vi "16_SynchronizedMeasurements.vi"() -> ()   [LabVIEW 2014]
uses:
  SwabianInstruments.TimeTagger
panel:
  out "FileWriter files":string[](array[string])
  out "First timestamp\ndifference":dbl[unit] format="%#.2g"
  out "Time-tag display":T1(graph)
  out "all time-tags\nidentical?":bool
  in  "Start synchronously if available":bool=TRUE
  in  "Use SynchronizedMeasurements":bool=TRUE
  # "This example demonstrates the SynchronizedMeasurements class. The time-tag stream is investigated by a TimeTagStream measurement and simultaneously dumped by a FileWriter measurement. Afterward, the resulting time-tag streams are compared.\n\nSynchronizedMeasurements ensures that both sub-measurements, TimeTagStream and FileWriter, process the very same set of time-tags. It can be activated/deactivated by the \"Use SynchronizedMeasurements\" control. Even with SynchronizedMeasurements, the sub-measurements can be controlled individually (use \"start synchronously if available\" to toggle behavior.\n\nSynchronizedMeasurements has an important impact on the FileWriter: It deactivates the autostart behavior. Without SynchronizedMeasurements, autostart + startFor results in two FileWriter data files, dump.1.ttbin and dump.2.ttbin."
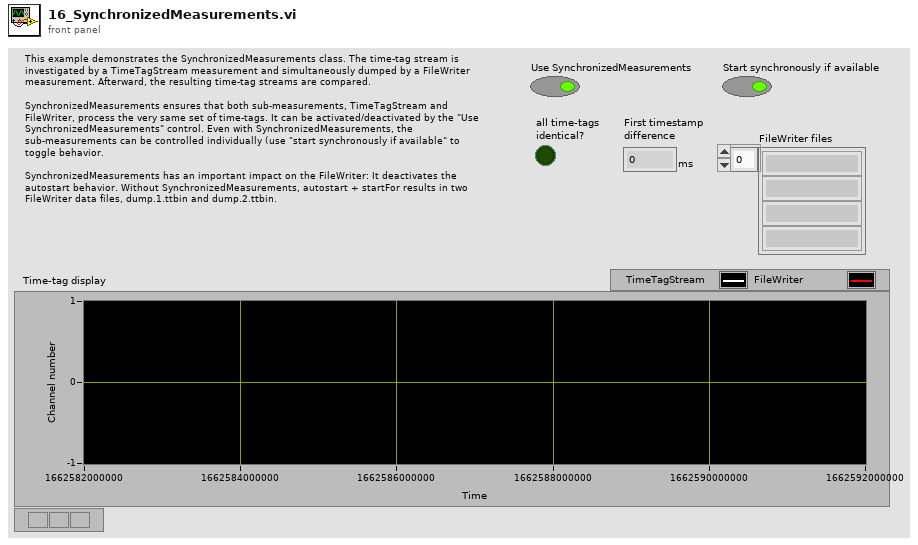
[diagram p1: front panel]
types:
  T1 = cluster{"getTimestamps":i64[], "getChannels":i32[]}[]
  T2 = cluster{"getTimestamps":i64[], "getChannels":i32[]}
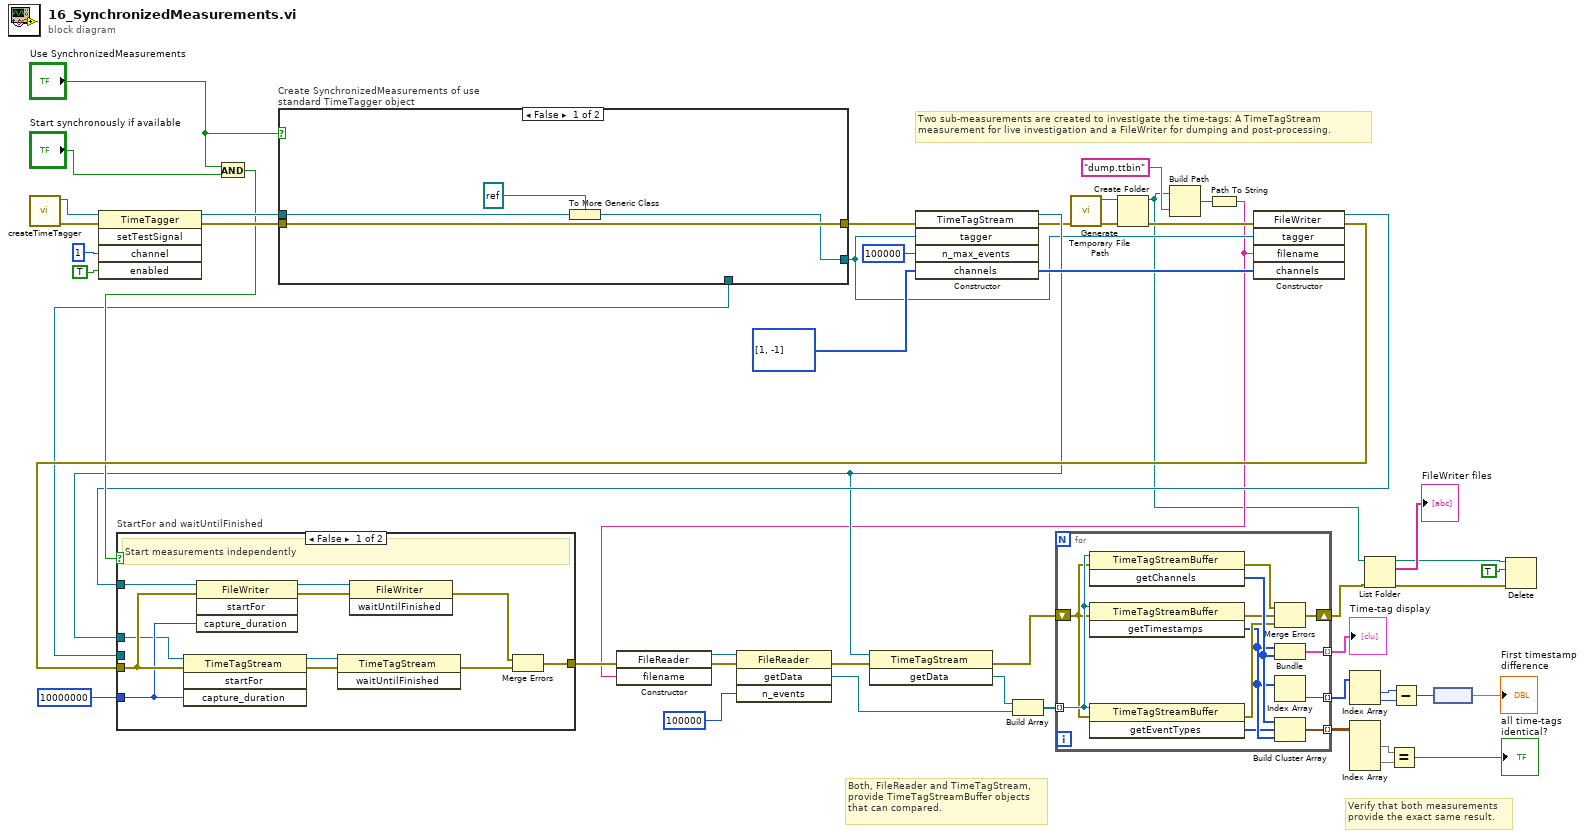
[diagram p0: block diagram]
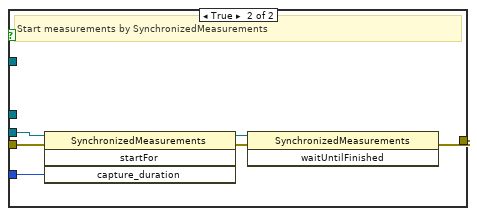
[diagram p2: hidden frame]
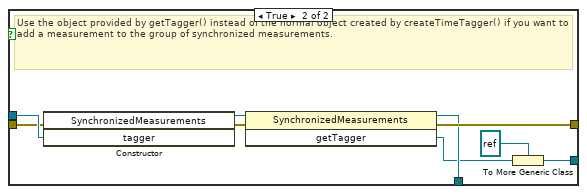
[diagram p3: hidden frame]
diagram:
  # "Both, FileReader and TimeTagStream,\nprovide TimeTagStreamBuffer objects\nthat can compared."
  # "Verify that both measurements\nprovide the exact same result."
  # "Two sub-measurements are created to investigate the time-tags: A TimeTagStream\nmeasurement for live investigation and a FileWriter for dumping and post-processing."
  n1 = call "createTimeTagger.vi"() -> ("error out"=w45:errorcluster, "TimeTagger ref out"=w46:refnum<k24>)  [unwired: 10 in]
  n2 = invoke class="TimeTagger" method="setTestSignal"(reference=w46, error in=w45, "channel"=1, "enabled"=TRUE) -> (reference out=w49:refnum<k24>, error out=w48:errorcluster)  [unwired: 1 in, 3 out]
  n3 = And(x="Use SynchronizedMeasurements", y="Start synchronously if available") -> (x .and. y?=w43:bool)
  n4 = case "Create SynchronizedMeasurements of use standard TimeTagger object" shown="False" "Use SynchronizedMeasurements" {
    tunnel: [w52 w56] -> w14
    tunnel: [w55 w62] -> w50
    tunnel: w49 -> [w53 w61]
    tunnel: w48 -> [w55 w60]
    tunnel: [_ w59] -> w22
    frame False {
      n5 = To More Generic Class(target class=refnum<k24> refnum, reference=w53) -> (generic class reference=w52:refnum<k24>)
    }
    frame True {
      # "Use the object provided by getTagger() instead of the normal object created by createTimeTagger() if you want to add a measurement to the group of synchronized measurements."
      n6 = constructor class="SynchronizedMeasurements"(error in=w60, "tagger"=w61) -> (reference out=w64:refnum<k24>, error out=w63:errorcluster)  [unwired: 2 in, 2 out]
      n7 = invoke class="SynchronizedMeasurements" method="getTagger"(reference=w64, error in=w63) -> (reference out=w59:refnum<k24>, error out=w62:errorcluster, "getTagger"=w58:refnum<k24>)  [unwired: 1 in]
      n8 = To More Generic Class(target class=refnum<k24> refnum, reference=w58) -> (generic class reference=w56:refnum<k24>)
    }
  }
  n9 = constructor class="TimeTagStream"(error in=w50, "tagger"=w14, "n_max_events"=u64 100000, "channels"=i32[] [1, -1]) -> (reference out=w20:refnum<k24>, error out=w5:errorcluster, "channels"=w23:i32[])  [unwired: 2 in, 3 out]
  n10 = call <vilib>:"Generate Temporary File Path.vi"("error in (no error)"=w5) -> ("error out"=w7:errorcluster, "Unique Temporary File Path"=w6:path)  [unwired: 9 in]
  n11 = Create Folder(path (use dialog)=w6, error in=w7) -> (created path=w1:path, error out=w4:errorcluster)  [unwired: 1 in, 1 out]
  n12 = Build Path(base path=w1, name or relative path="dump.ttbin") -> (appended path=w3:path)
  n13 = Path To String(path=w3) -> (string=w2:string)
  n14 = constructor class="FileWriter"(error in=w4, "tagger"=w14, "filename"=w2, "channels"=w23) -> (reference out=w41:refnum<k24>, error out=w47:errorcluster)  [unwired: 2 in, 4 out]
  n15 = case "StartFor and waitUntilFinished" shown="False" w43 {
    tunnel: w47 -> [w71 w81]
    tunnel: w22 -> [_ w80]
    tunnel: [w67 w77] -> w18
    tunnel: i64 10000000 ("capture_duration") -> [w70 w76]
    tunnel: w20 -> [w65 _]
    tunnel: w41 -> [w66 _]
    frame False {
      # "Start measurements independently"
      n16 = invoke class="TimeTagStream" method="startFor"(reference=w65, error in=w71, "capture_duration"=w70) -> (reference out=w73:refnum<k24>, error out=w72:errorcluster)  [unwired: 1 in, 2 out]
      n17 = invoke class="FileWriter" method="startFor"(reference=w66, error in=w71, "capture_duration"=w70) -> (reference out=w75:refnum<k24>, error out=w74:errorcluster)  [unwired: 1 in, 2 out]
      n18 = invoke class="TimeTagStream" method="waitUntilFinished"(reference=w73, error in=w72) -> (error out=w68:errorcluster)  [unwired: 1 in, 2 out]
      n19 = invoke class="FileWriter" method="waitUntilFinished"(reference=w75, error in=w74) -> (error out=w69:errorcluster)  [unwired: 1 in, 2 out]
      n20 = Merge Errors(w69, w68) -> (w67:errorcluster)
    }
    frame True {
      # "Start measurements by SynchronizedMeasurements"
      n21 = invoke class="SynchronizedMeasurements" method="startFor"(reference=w80, error in=w81, "capture_duration"=w76) -> (reference out=w79:refnum<k24>, error out=w78:errorcluster)  [unwired: 1 in, 2 out]
      n22 = invoke class="SynchronizedMeasurements" method="waitUntilFinished"(reference=w79, error in=w78) -> (error out=w77:errorcluster)  [unwired: 1 in, 2 out]
    }
  }
  n23 = constructor class="FileReader"(error in=w18, "filename"=w2) -> (reference out=w40:refnum<k24>, error out=w39:errorcluster)  [unwired: 2 in, 2 out]
  n24 = invoke class="FileReader" method="getData"(reference=w40, error in=w39, "n_events"=u64 100000) -> (error out=w16:errorcluster, "getData"=w31:refnum<k24>)  [unwired: 1 in, 2 out]
  n25 = invoke class="TimeTagStream" method="getData"(reference=w20, error in=w16) -> (error out=w15:errorcluster, "getData"=w38:refnum<k24>)  [unwired: 1 in, 1 out]
  n26 = Build Array(w38, w31) -> (w37:refnum<k24>[])
  n27 = for {
    tunnel: w37 -> [w93] mode=indexing
    tunnel: [w92] -> w36 mode=indexing
    tunnel: [w91] -> w32 mode=indexing
    shift-right: [w85] -> w11
    shift-left: w15 -> [w89]
    tunnel: [w83] -> w30 mode=indexing
    n28 = invoke class="TimeTagStreamBuffer" method="getChannels"(reference=w93, error in=w89) -> (error out=w86:errorcluster, "getChannels"=w90:i32[])  [unwired: 1 in, 1 out]
    n29 = invoke class="TimeTagStreamBuffer" method="getTimestamps"(reference=w93, error in=w89) -> (error out=w87:errorcluster, "getTimestamps"=w84:i64[])  [unwired: 1 in, 1 out]
    n30 = invoke class="TimeTagStreamBuffer" method="getEventTypes"(reference=w93, error in=w89) -> (error out=w88:errorcluster, "getEventTypes"=w82:u8[])  [unwired: 1 in, 1 out]
    n31 = Merge Errors(w86, w87, w88) -> (w85:errorcluster)
    n32 = Bundle("getTimestamps"=w84, "getChannels"=w90) -> (w91:T2)  [unwired: 1 in]
    n33 = Index Array(array=w84) -> (element=w83:i64)  [unwired: 1 in]
    n34 = Build Cluster Array(w90, w82, w84) -> (w92:cluster{i32, u8, i64}[])
  }
  "Time-tag display" <- w32
  n35 = Index Array(array=w30) -> (element #1=w29:i64, element #2=w28:i64)  [unwired: 2 in]
  n36 = Index Array(array=w36) -> (element #1=w35:cluster{i32, u8, i64}[], element #2=w34:cluster{i32, u8, i64}[])  [unwired: 4 in]
  n37 = List Folder(path=w1, error in=w11) -> (path out=w9:path, filenames=→"FileWriter files":string[], error out=w10:errorcluster)  [unwired: 2 in, 1 out]
  n38 = Equal?(x=w35, y=w34) -> (x = y?=→"all time-tags\nidentical?":bool)
  n39 = Subtract(x=w29, y=w28) -> (x-y=w27:i64)
  n40 = node(w27) -> (→"First timestamp\ndifference":dbl[unit])
  n41 = Delete(path (use dialog)=w9, entire hierarchy (F)=TRUE, error in=w10) -> ()  [unwired: 2 in, 3 out]
